vi "GDSProject_GetLibraryMemberRealAndVirtualPath.vi"(1 "LibraryItem":refnum<vi>, 5 "error in (no error)":errorcluster) -> (15 "LibraryItemRealPath":path, 17 "LibraryItemVirtualPath":path, 18 "VirtualFolderScope":T1(array[ring]), 19 "error out":errorcluster)   [LabVIEW 2020]
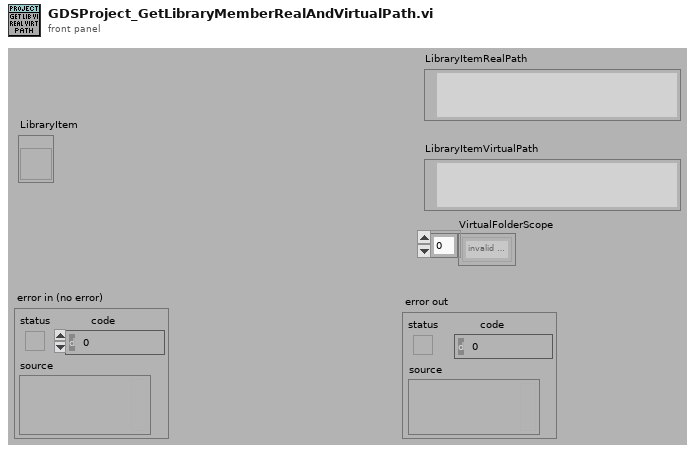
[diagram p1: front panel]
types:
  T1 = enum32{"invalid scope", "public", "private", "protected", "community"}[]
  T2 = enum32{"invalid scope", "public", "private", "protected", "community"}
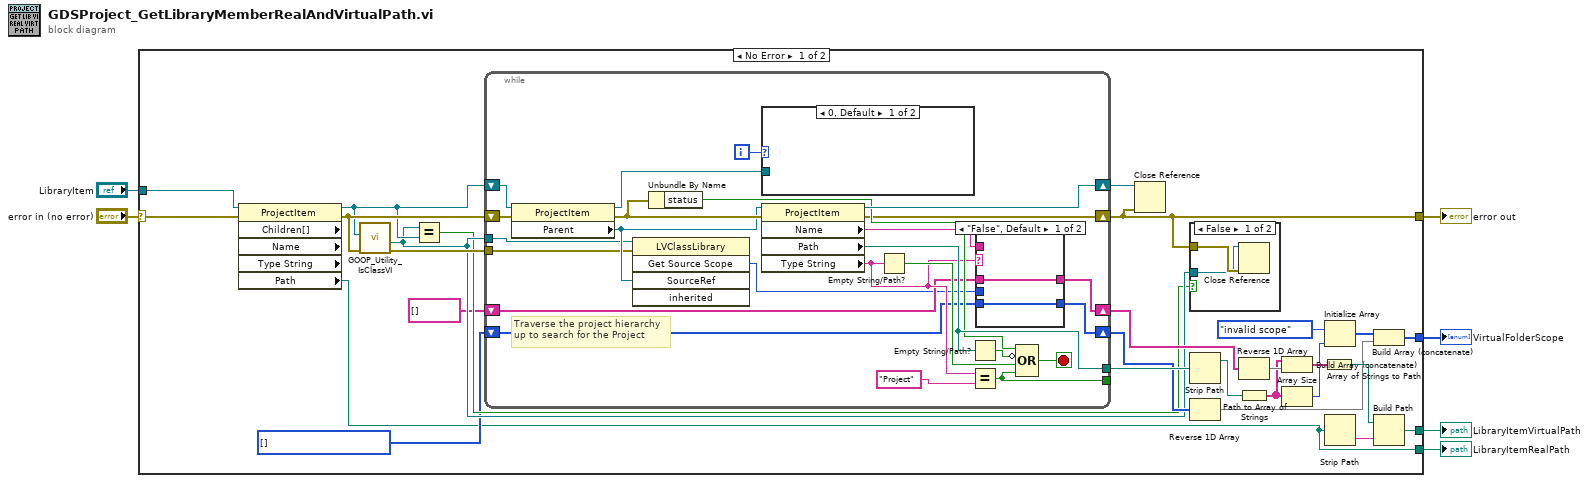
[diagram p0: block diagram]
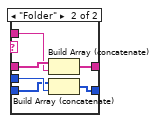
[diagram p3: hidden frame]
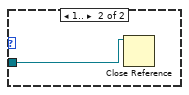
[diagram p4: hidden frame]
diagram:
  n1 = case shown="No Error" "error in (no error)" {
    selector: "error in (no error)" -> [w32 w69]
    tunnel: [w33 w69] -> w5
    tunnel: "LibraryItem" -> [w31 _]
    tunnel: [w13 _] -> w2
    tunnel: [w16 _] -> w3
    tunnel: [w7 _] -> w1
    frame No Error {
      w18 = T1 [] items=["invalid scope", "public", "private", "protected", "community"]
      n2 = property class="ProjectItem" props=["Children[]", "Name", "Type String", "Path"](reference=w31, error in=w32) -> (reference out=w29:refnum<vi>, error out=w30:errorcluster, "Path"=w16:path)  [unwired: 3 out]
      n3 = call "GOOP_Utility_IsClassVI.vi"("error in (no error)"=w30, "ProjectItem"=w29) -> ("error out"=w21:errorcluster, "ClassItem(If Found)"=w20:refnum<vi>)  [unwired: 4 in, 4 out]
      n4 = Equal?(x=w20, y=w29) -> (x = y?=w19:bool)
      n5 = while {
        shift-right: [w58] -> w25
        shift-left: w29 -> [w59]
        tunnel: [w51] -> w27
        tunnel: [w52] -> _
        shift-right: [w47] -> w33
        shift-left: w30 -> [w41]
        shift-right: [w44] -> w24
        shift-left: string[] [] -> [w45]
        shift-right: [w39] -> w22
        shift-left: w18 -> [w38]
        tunnel: w20 -> [w37]
        tunnel: w21 -> [w36]
        i -> [w54]
        stop <- w57 stop-if-true
        # "Traverse the project hierarchy\nup to search for the Project"
        n6 = property class="ProjectItem"(reference=w59, error in=w41) -> (reference out=w55:refnum<vi>, error out=w48:errorcluster, "Parent"=w42:refnum<vi>)
        n7 = invoke class="LVClassLibrary" method="Get Source Scope"(reference=w37, error in=w36, "SourceRef"=w42) -> ("GetSourceScope"=w40:T2)  [unwired: 2 in, 4 out]
        n8 = Unbundle By Name(w48) -> ("status"=w50:bool)
        n9 = case shown="0, Default" w54 {
          tunnel: w55 -> [_ w68]
          frame 0, Default {
          }
          frame 1.. {
            n10 = Close Reference(reference=w68) -> ()  [unwired: 1 in, 1 out]
          }
        }
        n11 = property class="ProjectItem"(reference=w42, error in=w48) -> (reference out=w58:refnum<vi>, error out=w47:errorcluster, "Name"=w43:string, "Path"=w51:path, "Type String"=w46:string)
        n12 = Empty String/Path?(string/path=w46) -> (empty?=w53:bool)
        n13 = Empty String/Path?(string/path=w51) -> (empty?=w49:bool)
        n14 = Equal?(x=w46, y="Project") -> (x = y?=w52:bool)
        n15 = case shown="\"False\", Default" w46 {
          tunnel: w45 -> [w61 w67]
          tunnel: [w61 w66] -> w44
          tunnel: w43 -> [_ w65]
          tunnel: w40 -> [_ w64]
          tunnel: [w60 w63] -> w39
          tunnel: w38 -> [w60 w62]
          frame "False", Default {
          }
          frame "Folder" {
            n16 = Build Array (concatenate)(w67, w65) -> (w66:string[])
            n17 = Build Array (concatenate)(w62, w64) -> (w63:T1)
          }
        }
        n18 = Compound Arithmetic op=OR(w50, invert w49, w53, w52) -> (w57:bool)
      }
      n19 = Close Reference(reference=w25, error in (no error)=w33) -> ()  [unwired: 1 out]
      n20 = case shown="False" w19 {
        tunnel: w33 -> [w35 _]
        tunnel: w20 -> [w34 _]
        frame False {
          n21 = Close Reference(reference=w34, error in (no error)=w35) -> ()  [unwired: 1 out]
        }
        frame True {
        }
      }
      n22 = Strip Path(path=w27) -> (stripped path=w26:path)  [unwired: 1 out]
      n23 = Reverse 1D Array(array=w22) -> (reversed array=w9:T1)
      n24 = Reverse 1D Array(array=w24) -> (reversed array=w23:string[])
      n25 = Path to Array of Strings(0:w26) -> (2:w12:string[])  [unwired: 1 out]
      n26 = Build Array (concatenate)(w12, w23) -> (w28:string[])
      n27 = Array Size(array=w12) -> (size(s)=w11:i32)
      n28 = Array of Strings to Path(0:w28) -> (2:w14:path)  [unwired: 1 in]
      n29 = Initialize Array(T2."invalid scope" ("GetSourceScope"), w11) -> (w10:T1)
      n30 = Strip Path(path=w16) -> (name=w15:string)  [unwired: 1 out]
      n31 = Build Array (concatenate)(w10, w9) -> (w7:T1)
      n32 = Build Path(base path=w14, name or relative path=w15) -> (appended path=w13:path)
    }
    frame Error {
    }
  }
  "error out" <- w5
  "LibraryItemRealPath" <- w3
  "LibraryItemVirtualPath" <- w2
  "VirtualFolderScope" <- w1
